vi "编码输出.vi"(8 "error in (no error)":errorcluster, 11 "SingleStepTestV3输入":refnum<class "SingleStepTestV3.lvclass">) -> (0 "error out":errorcluster)   [LabVIEW 2016, in "SingleStepTestV3.lvlib" / "SingleStepTestV3.lvclass"]
uses:
  SingleStepTestV3.lvclass
  SingleStepTestV3.lvclass/SingleStepTestV3.ctl
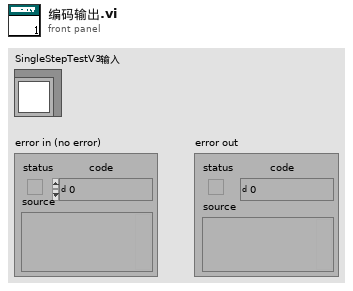
[diagram p1: front panel]
types:
  T1 = typedef "SingleStepTestV3.lvlib/SingleStepTestV3.lvclass/仪器版本.ctl" = enum16{"A版", "B版", "A1版"}
  T2 = typedef "SingleStepTestV3.lvlib/SingleStepTestV3.lvclass/State Data.ctl" = cluster{"data":u16[], "仪器版本":T1}
  T3 = typedef "SingleStepTestV3.lvclass/外设选择2.ctl" = cluster{"V9-1":bool, "V9-2":bool, "顺时针":bool, "逆时针":bool}
  T4 = typedef "SingleStepTestV3.lvclass/注射泵操作.ctl" = enum32{"复位", "注入", "注出", "等待"}
  T5 = typedef "SingleStepTestV3.lvclass/控温操作.ctl" = cluster{"氨氮控温":bool, "消解":bool, "恒温":bool, "降温":bool}
  T6 = typedef "SingleStepTestV3.lvclass/外设选择.ctl" = cluster{"蠕动泵":bool, "电磁阀1":bool, "电磁阀2":bool, "慢速":bool}
  T7 = typedef "SingleStepTestV3.lvclass/灯选择.ctl" = enum32{"未选择", "365", "520", "660", "氙灯/紫灯"}
  T8 = typedef "SingleStepTestV3.lvclass/ADC选择.ctl" = enum32{"未选择", "ADC365", "ADC520", "ADC660", "光谱仪"}
  T9 = typedef "SingleStepTestV3.lvclass/阀口操作.ctl" = enum32{"未选择", "V1", "V2", "V3", "V4", "V5", "V6", "V7", "V8", "V9", "V10", "V11", "V12"}
  T10 = typedef "SingleStepTestV3.lvclass/项目输入.ctl" = u16
  T11 = typedef "SingleStepTestV3.lvclass/数值输入.ctl" = i16
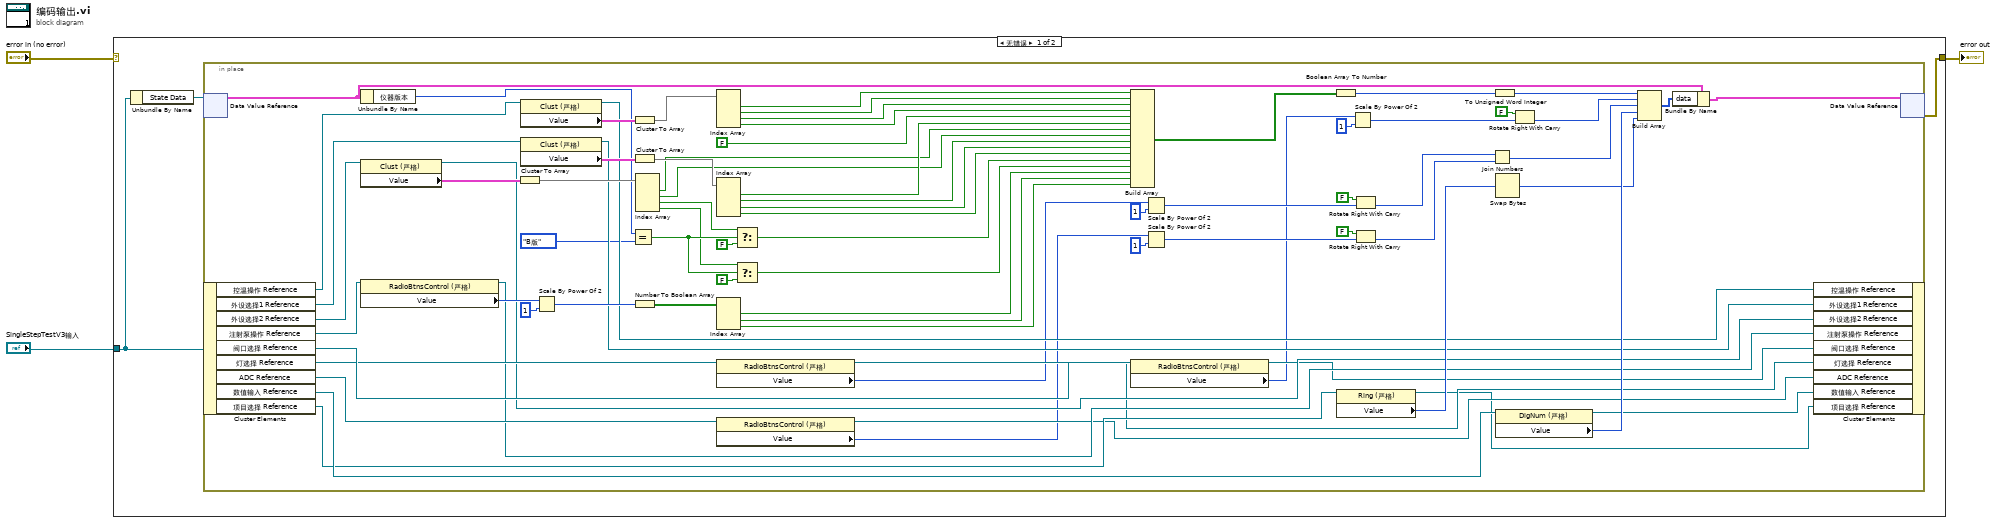
[diagram p0: block diagram]
diagram:
  n1 = case shown="无错误" "error in (no error)" {
    selector: "error in (no error)" -> [_ w83]
    tunnel: "SingleStepTestV3输入" -> [w5 _]
    tunnel: [w4 w83] -> w2
    frame No Error {
      n2 = Unbundle By Name(w5) -> ("State Data"=w6:refnum<data-value>)
      n3 = in-place {
        n4 = in-place-dvr #1(w6) -> (w19:T2)  [unwired: 1 out]
        n5 = in-place-cluster #2(w5) -> ("控温操作 Reference"=w82:refnum<vi>, "外设选择1 Reference"=w66:refnum<vi>, "外设选择2 Reference"=w65:refnum<vi>, "注射泵操作 Reference"=w64:refnum<vi>, "阀口选择 Reference"=w54:refnum<vi>, "灯选择 Reference"=w52:refnum<vi>, "ADC Reference"=w51:refnum<vi>, "数值输入 Reference"=w48:refnum<vi>, "项目选择 Reference"=w47:refnum<vi>)
        n6 = Unbundle By Name(w19) -> ("仪器版本"=w18:T1)
        n7 = property class="Clust (严格)"(reference=w65) -> (reference out=w35:refnum<vi>, "Value"=w79:T3)  [unwired: 1 in, 1 out]
        n8 = property class="RadioBtnsControl (严格)"(reference=w64) -> (reference out=w34:refnum<vi>, "Value"=w76:T4)  [unwired: 1 in, 1 out]
        n9 = Cluster To Array(cluster=w79) -> (array=w74:bool[])
        n10 = property class="Clust (严格)"(reference=w82) -> (reference out=w37:refnum<vi>, "Value"=w81:T5)  [unwired: 1 in, 1 out]
        n11 = property class="Clust (严格)"(reference=w66) -> (reference out=w36:refnum<vi>, "Value"=w80:T6)  [unwired: 1 in, 1 out]
        n12 = Scale By Power Of 2(n=w76, x=u8 1) -> (x*2^n=w77:u8)
        n13 = Equal?(x=w18, y=仪器版本."B版") -> (x = y?=w13:bool)
        n14 = Cluster To Array(cluster=w81) -> (array=w72:bool[])
        n15 = Cluster To Array(cluster=w80) -> (array=w73:bool[])
        n16 = Number To Boolean Array(number=w77) -> (Boolean array=w75:bool[])
        n17 = Index Array(array=w74) -> (element #1=w59:bool, element #2=w58:bool, element #3=w16:bool, element #4=w12:bool)  [unwired: 4 in]
        n18 = Index Array(array=w72) -> (element #1=w71:bool, element #2=w70:bool, element #3=w69:bool, element #4=w68:bool)  [unwired: 4 in]
        n19 = Index Array(array=w73) -> (element #1=w63:bool, element #2=w62:bool, element #3=w61:bool, element #4=w60:bool)  [unwired: 4 in]
        n20 = Index Array(array=w75) -> (element #1=w57:bool, element #2=w56:bool, element #3=w55:bool)  [unwired: 3 in]
        n21 = property class="RadioBtnsControl (严格)"(reference=w52) -> (reference out=w32:refnum<vi>, "Value"=w20:T7)  [unwired: 1 in, 1 out]
        n22 = property class="RadioBtnsControl (严格)"(reference=w51) -> (reference out=w31:refnum<vi>, "Value"=w21:T8)  [unwired: 1 in, 1 out]
        n23 = Select(t=w16, s=w13, f=FALSE) -> (s? t:f=w15:bool)
        n24 = Select(t=w12, s=w13, f=FALSE) -> (s? t:f=w11:bool)
        n25 = Build Array(w71, w70, w69, w68, FALSE, w63, w59, w58, w62, w61, w60, w15, w11, w57, w56, w55) -> (w43:bool[])
        n26 = property class="RadioBtnsControl (严格)"(reference=w54) -> (reference out=w33:refnum<vi>, "Value"=w26:T9)  [unwired: 1 in, 1 out]
        n27 = Scale By Power Of 2(n=w20, x=u8 1) -> (x*2^n=w44:u8)
        n28 = Scale By Power Of 2(n=w21, x=u8 1) -> (x*2^n=w45:u8)
        n29 = Boolean Array To Number(Boolean array=w43) -> (number=w42:u32)
        n30 = property class="Ring (严格)"(reference=w47) -> (reference out=w29:refnum<vi>, "Value"=w46:T10)  [unwired: 1 in, 1 out]
        n31 = Scale By Power Of 2(n=w26, x=u16 1) -> (x*2^n=w7:u16)
        n32 = Rotate Right With Carry(2:w44, 3:FALSE ("进位")) -> (0:w25:u8)  [unwired: 1 out]
        n33 = Rotate Right With Carry(2:w45, 3:FALSE ("进位")) -> (0:w23:u8)  [unwired: 1 out]
        n34 = Join Numbers(hi=w25, lo=w23) -> ((hi.lo)=w41:u16)
        n35 = To Unsigned Word Integer(number=w42) -> (unsigned 16bit integer=w38:u16)
        n36 = Swap Bytes(anything=w46) -> (byte swapped=w39:T10)
        n37 = property class="DigNum (严格)"(reference=w48) -> (reference out=w30:refnum<vi>, "Value"=w40:T11)  [unwired: 1 in, 1 out]
        n38 = Rotate Right With Carry(2:w7, 3:FALSE ("进位")) -> (0:w8:u16)  [unwired: 1 out]
        n39 = Build Array(w38, w8, w41, w40, w39) -> (w27:T10[])
        n40 = Bundle By Name(cluster=w19, "data"=w27) -> (w28:T2)
        n41 = in-place-cluster #2("控温操作 Reference"=w37, "外设选择1 Reference"=w36, "外设选择2 Reference"=w35, "注射泵操作 Reference"=w34, "阀口选择 Reference"=w33, "灯选择 Reference"=w32, "ADC Reference"=w31, "数值输入 Reference"=w30, "项目选择 Reference"=w29) -> ()  [unwired: 1 out]
        n42 = in-place-dvr #1(w28) -> (w4:errorcluster)  [unwired: 1 out]
      }
    }
    frame Error {
    }
  }
  "error out" <- w2
